vi "edittest load step.vi"(7 "incoming UID (\"\")":string, 8 "error in (no error)":errorcluster, 9 "POST Step Config (empty)":T1, 10 "sxTestId or ixStep (\"\")":string, 11 "Connection Refnum":T2) -> (0 "error out":errorcluster, 1 "Template Keys":T1, 2 "sxTestId":string, 3 "Connection Refnum":T2)   [LabVIEW 2011]
uses:
  Addons/internet/utils/keyedarr.llb/Keyed Array.ctl
  SI.LIB/ODBC/SQL Controls/Connection Refnum.ctl
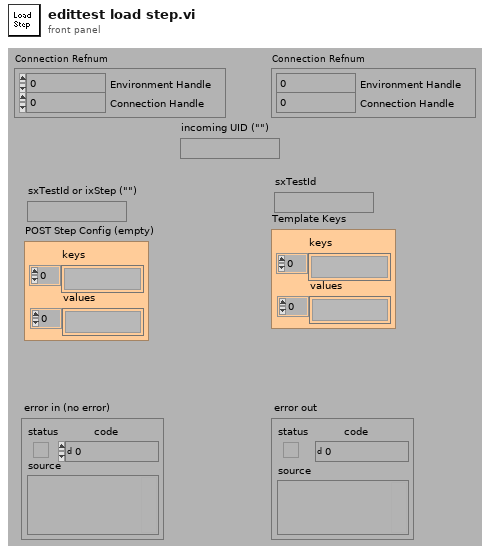
[diagram p1: front panel]
types:
  T1 = typedef "Keyed Array.ctl" = cluster{"keys":string[], "values":string[]}
  T2 = typedef "Connection Refnum.ctl" = cluster{"Environment Handle":i32, "Connection Handle":i32}
  T3 = typedef "Step Record.ctl" = cluster{"ixStep":i32, "sxSequenceId":string, "sxTestId":string, "iIndex":i32, "iRepeat":i32, "iQuickMode":i32, "sTag":string, "sDatasheetsCSV":string, "bConfiguration":string}
  T4 = typedef "Test Record.ctl" = cluster{"ixTest":i32, "sxTestId":string, "sVersion":string, "sDriverTypes":string[], "sDescription":string, "iQuickMode":i32}
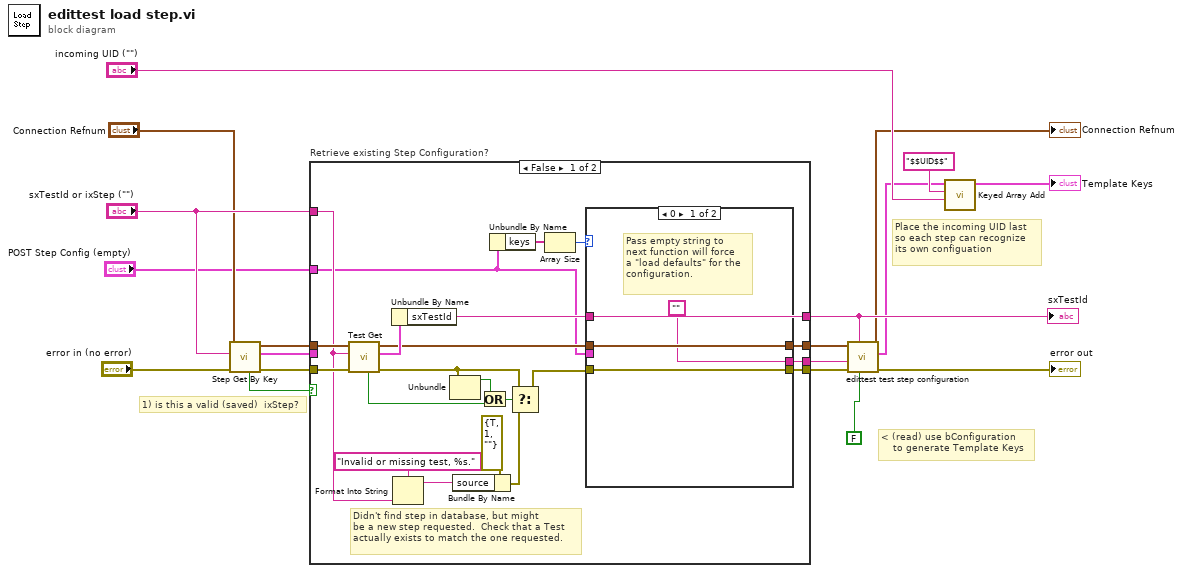
[diagram p0: block diagram]
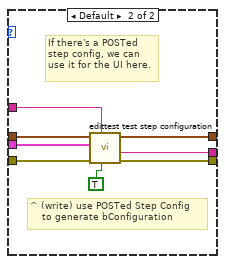
[diagram p2: hidden frame]
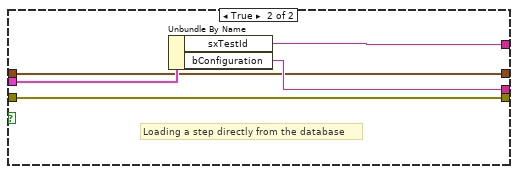
[diagram p3: hidden frame]
diagram:
  # "< (read) use bConfiguration\n    to generate Template Keys"
  # "Place the incoming UID last\nso each step can recognize\nits own configuation"
  # "1) is this a valid (saved)  ixStep?"
  n1 = call "Step Get By Key.vi"("error in (no error)"="error in (no error)", "ixStep"="sxTestId or ixStep (\"\")", "Connection Refnum"="Connection Refnum") -> ("error out"=w9:errorcluster, "Step Record"=w14:T3, "Connection Refnum"=w10:T2, "Data Present"=w12:bool)  [unwired: 5 out]
  n2 = case "Retrieve existing Step Configuration?" shown="False" w12 {
    tunnel: w14 -> [_ w56]
    tunnel: [w24 w55] -> w5
    tunnel: [w26 w54] -> w13
    tunnel: "sxTestId or ixStep (\"\")" -> [w29 _]
    tunnel: w10 -> [w40 w52]
    tunnel: w9 -> [w39 w53]
    tunnel: [w27 w53] -> w7
    tunnel: "POST Step Config (empty)" -> [w22 _]
    tunnel: [w23 w52] -> w4
    frame False {
      # "Didn't find step in database, but might\nbe a new step requested.  Check that a Test\nactually exists to match the one requested."
      n3 = call "Test Get.vi"("error in (no error)"=w39, "Test_ID"=w29, "Connection Refnum"=w40) -> ("error out"=w34:errorcluster, "Test Record"=w38:T4, "Connection Refnum"=w25:T2, "Data Present"=w36:bool)  [unwired: 5 out]
      n4 = Unbundle By Name(w38) -> ("sxTestId"=w24:string)
      n5 = Format Into String(format string="Invalid or missing test, %s." ("source"), w29) -> (resulting string=w30:string)  [unwired: 2 in, 1 out]
      n6 = Unbundle(w34) -> ("status"=w37:bool)  [unwired: 2 out]
      n7 = Bundle By Name(cluster=errorcluster {"status"=TRUE, "code"=1, "source"=""} ("f"), "source"=w30) -> (w32:errorcluster)
      n8 = Or(x=w37, y=w36) -> (x .or. y?=w35:bool)
      n9 = Unbundle By Name(w22) -> ("keys"=w21:string[])
      n10 = Select(t=w34, s=w35, f=w32) -> (s? t:f=w28:errorcluster)
      n11 = Array Size(array=w21) -> (size(s)=w20:i32)
      n12 = case shown="0" w20 {
        tunnel: w28 -> [w42 w51]
        tunnel: [w42 w50] -> w27
        tunnel: ["" w49] -> w26
        tunnel: w25 -> [w43 w47]
        tunnel: w24 -> [_ w46]
        tunnel: [w43 w45] -> w23
        tunnel: w22 -> [_ w44]
        frame 0 {
          # "Pass empty string to\nnext function will force\na \"load defaults\" for the\nconfiguration."
        }
        frame Default {
          # "^ (write) use POSTed Step Config\n    to generate bConfiguration"
          # "If there's a POSTed\nstep config, we can\nuse it for the UI here."
          n13 = call "edittest test step configuration.vi"("Write? (f)"=TRUE, "sxTestId (\"\")"=w46, "error in (no error)"=w51, "POSTed Step Config (to Write to bConfiguration)\nOR\nTemplate Keys (empty)"=w44, "Connection Refnum"=w47) -> ("error out"=w50:errorcluster, "bConfiguration"=w49:string, "Connection Refnum"=w45:T2)  [unwired: 2 in, 2 out]
        }
      }
    }
    frame True {
      # "Loading a step directly from the database"
      n14 = Unbundle By Name(w56) -> ("sxTestId"=w55:string, "bConfiguration"=w54:string)
    }
  }
  "sxTestId" <- w5
  n15 = call "edittest test step configuration.vi"("Write? (f)"=FALSE, "sxTestId (\"\")"=w5, "error in (no error)"=w7, "bConfiguration (to Read for Template Keys) (\"\")"=w13, "Connection Refnum"=w4) -> ("error out"=→"error out":errorcluster, "Template Keys"=w1:T1, "Connection Refnum"=→"Connection Refnum":T2)  [unwired: 2 in, 2 out]
  n16 = call "Keyed Array Add.vi"("value"="incoming UID (\"\")", "key"="$$UID$$", "array in"=w1) -> ("array out"=→"Template Keys":T1)  [unwired: 1 in, 3 out]
